vi "LoopControl.vi"(8 "error IO":errorcluster, 11 "QueueCluste":T1) -> (3 "error IO 2":errorcluster)   [LabVIEW 2017, in "libVariable.lvlib" / "LibFunction.lvlib"]
uses:
  LibFunction.lvlib
  controls/QueueControl.ctl
  controls/CommandQueue.ctl
  <vilib>/Platform/TimedLoop/XDataNode/timing_clust.ctl
  <vilib>/Platform/TimedLoop/XDataNode/nitl_modes.ctl
  <vilib>/Platform/TimedLoop/XDataNode/wakeup.ctl
  controls/stateAutoMode.ctl
  controls/stateModeDevice.ctl
  controls/gcodeArray.ctl
  global/globalStartAuto.vi
  <vilib>/Platform/TimedLoop/XDataNode/XDataNode.xnode
  <vilib>/Platform/TimedLoop/XDataNode/XDNodeRunTimeDep.lvlib
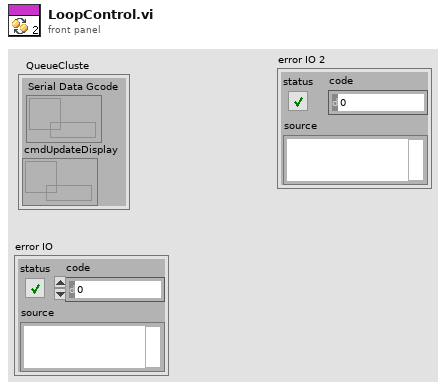
[diagram p1: front panel]
types:
  T1 = typedef "QueueControl.ctl" = cluster{"Serial Data Gcode":refnum<queue>, "cmdUpdateDisplay":refnum<queue>}
  T2 = typedef "stateAutoMode.ctl" = enum16{"init", "wait", "running", "end"}
  T3 = typedef "XDNodeRunTimeDep.lvlib/timing_clust.ctl" = cluster{"Expected End [f-1]":u64, "Actual End [f-1]":u64, "Finished Late? [f-1]":bool, "Expected End [i-1]":u64, "Actual End [i-1]":u64, "Finished Late? [i-1]":bool, "Expected Start [i]":u64, "Actual Start [i]":u64, "Expected Start [f]":u64, "Actual Start [f]":u64, "Source Name":string, "Structure Name":string, "Period":i64, "Deadline":i64, "Offset":i64, "Start":i64, "Priority":i32, "Timeout":i32, "Mode":T4, "Wakeup Reason":T5, "Error":errorcluster, "Source Type":string, "Secondary Source Type":string, "Global End Time":u64, "Global Start Time":u64, "Frame Duration":u64, "Iteration Duration":u64, "Assigned CPU":i32, "I/O Scan Engine Mode":u32}
  T4 = typedef "XDNodeRunTimeDep.lvlib/nitl_modes.ctl" = enum32{"No Change", "Process missed periods, maintain original phase", "Discard missed periods, maintain original phase", "Process missed periods, ignore original phase", "Discard missed periods, ignore original phase"}
  T5 = typedef "XDNodeRunTimeDep.lvlib/wakeup.ctl" = enum32{"Normal", "Aborted", "Asynchronous wakeup", "Timing source error", "Timed loop error", "Timeout"}
  T6 = typedef "stateModeDevice.ctl" = enum16{"Auto", "Menu", "WaitAutoFinish", "Config", "initAuto"}
  T7 = typedef "gcodeArray.ctl" = string[]
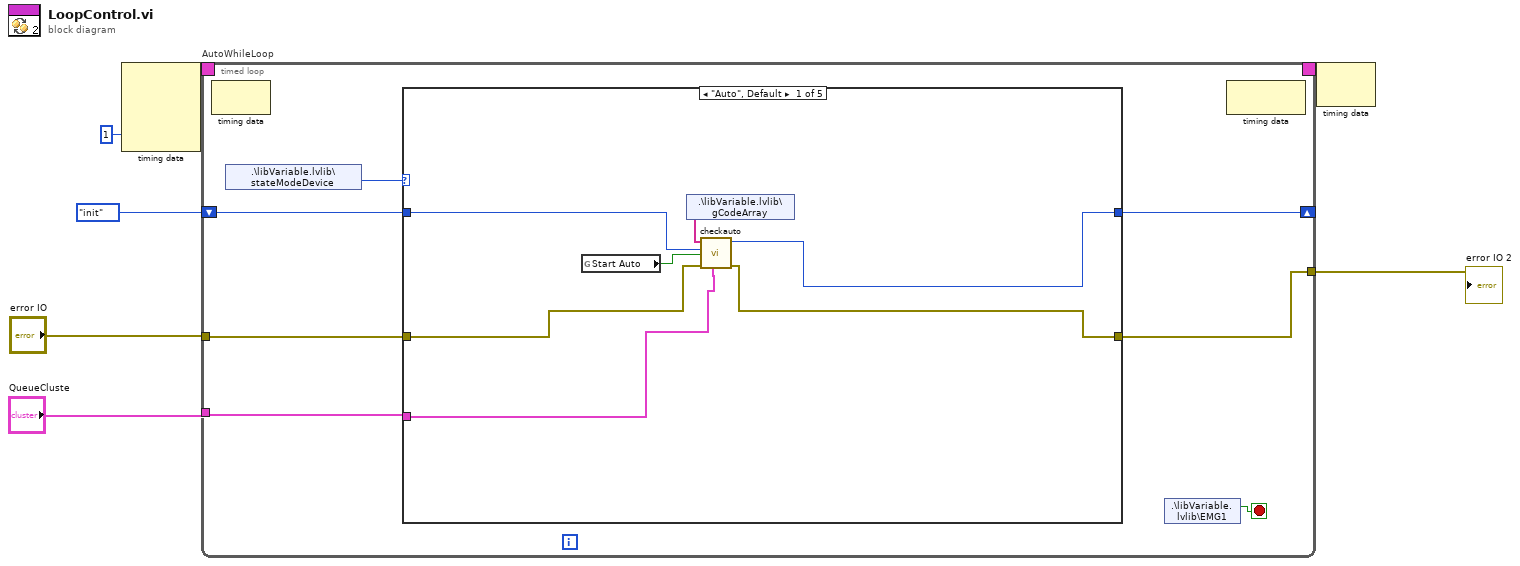
[diagram p0: block diagram]
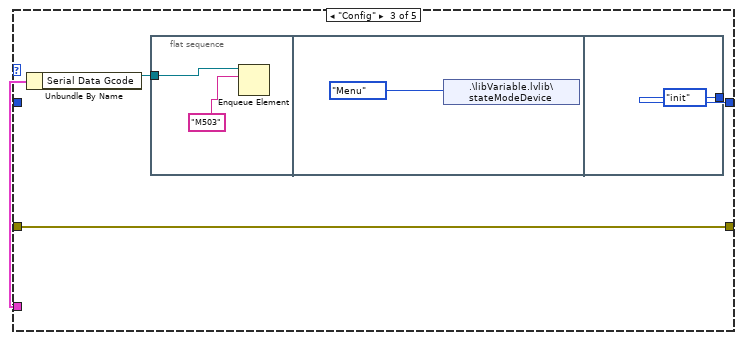
[diagram p3: hidden frame]
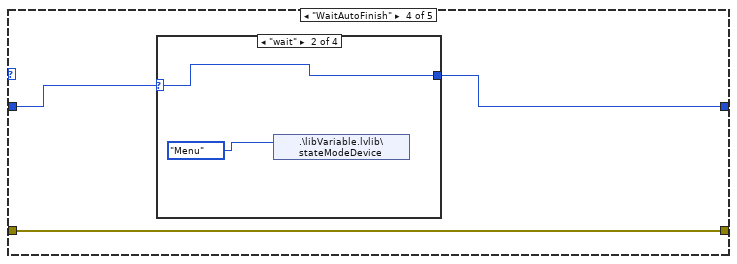
[diagram p4: hidden frame]
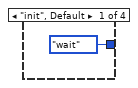
[diagram p5: hidden frame]
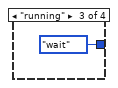
[diagram p6: hidden frame]
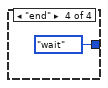
[diagram p7: hidden frame]
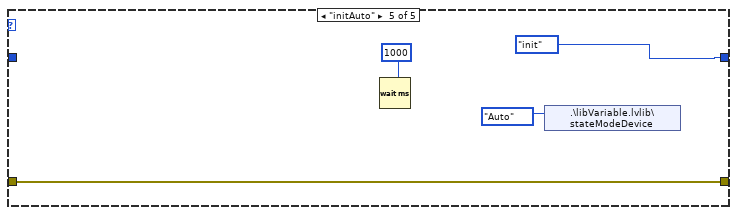
[diagram p8: hidden frame]
diagram:
  n1 = node-c288(1 ("Processor")) -> (w7:T3)  [unwired: 3 in]
  n2 = timed-loop "AutoWhileLoop" {
    shift-right: [w12] -> _
    shift-left: stateAutoMode."init" -> [w14]
    tunnel: "error IO" -> [w11]
    tunnel: "QueueCluste" -> [w13]
    tunnel: [w9] -> w1
    timing: w7 -> [_]
    timing-out: [_] -> w6
    stop <- w8 stop-if-true
    n3 = node-c288() -> ()  [unwired: 1 in, 1 out]
    n4 = shared-variable ".\\libVariable.lvlib\\stateModeDevice"() -> (w10:T6)  [unwired: 1 in, 1 out]
    n5 = case shown="\"Auto\", Default" w10 {
      tunnel: w14 -> [w19 w25 _ w34 _]
      tunnel: [w23 w25 w27 w36 stateAutoMode."init"] -> w12
      tunnel: w13 -> [w21 _ w29 _ _]
      tunnel: w11 -> [w17 w24 w26 w35 w45]
      tunnel: [w22 w24 w26 w35 w45] -> w9
      frame "Auto", Default {
        n6 = global read "globalStartAuto.vi" "Start Auto"() -> (w18:bool)
        n7 = shared-variable ".\\libVariable.lvlib\\gCodeArray"() -> (w20:T7)  [unwired: 1 in, 1 out]
        n8 = call "checkauto.vi"("G-Code Array"=w20, "stateAuto in"=w19, "Start Auto"=w18, "error in (no error)"=w17, "queue"=w21) -> ("stateAuto out"=w23:T2, "error out"=w22:errorcluster)  [unwired: 4 in]
      }
      frame "Menu" {
      }
      frame "Config" {
        n9 = Unbundle By Name(w29) -> ("Serial Data Gcode"=w28:refnum<queue>)
        n10 = flat-sequence {
          tunnel: w28 -> [w30]
          tunnel: [stateAutoMode."init"] -> w27
          frame #0 {
            n11 = Enqueue Element(queue=w30, element="M503") -> ()  [unwired: 2 in, 3 out]
          }
          frame #1 {
            n12 = shared-variable ".\\libVariable.lvlib\\stateModeDevice"(stateModeDevice."Menu" ("statusMode")) -> ()  [unwired: 1 in, 1 out]
          }
          frame #2 {
          }
        }
      }
      frame "WaitAutoFinish" {
        n13 = case shown="\"wait\"" w34 {
          selector: w34 -> [_ w39 _ _]
          tunnel: [stateAutoMode."wait" w39 stateAutoMode."wait" stateAutoMode."wait"] -> w36
          frame "init", Default {
          }
          frame "wait" {
            n14 = shared-variable ".\\libVariable.lvlib\\stateModeDevice"(stateModeDevice."Menu" ("statusMode")) -> ()  [unwired: 1 in, 1 out]
          }
          frame "running" {
          }
          frame "end" {
          }
        }
      }
      frame "initAuto" {
        n15 = Wait (ms)(milliseconds to wait=u32 1000) -> ()  [unwired: 1 out]
        n16 = shared-variable ".\\libVariable.lvlib\\stateModeDevice"(stateModeDevice."Auto" ("statusMode")) -> ()  [unwired: 1 in, 1 out]
      }
    }
    n17 = shared-variable ".\\libVariable.lvlib\\EMG1"() -> (w8:bool)  [unwired: 1 in, 1 out]
    n18 = node-c288() -> ()  [unwired: 1 in, 1 out]
  }
  "error IO 2" <- w1
  n19 = node-c288(w6) -> ()  [unwired: 1 out]
